vi "graphOnScreen.vi"(6 "Connect to loop iteration":i32, 8 "Time":dbl, 9 "332 Temp [K]":dbl, 10 "332 Temp Setpoint [K]":dbl, 11 "R(ohm)":dbl) -> (0 "T(t)":cluster{"X":dbl, "Y":dbl}[](graph), 3 "?":cluster{dbl, dbl}[](graph))   [LabVIEW 2012]
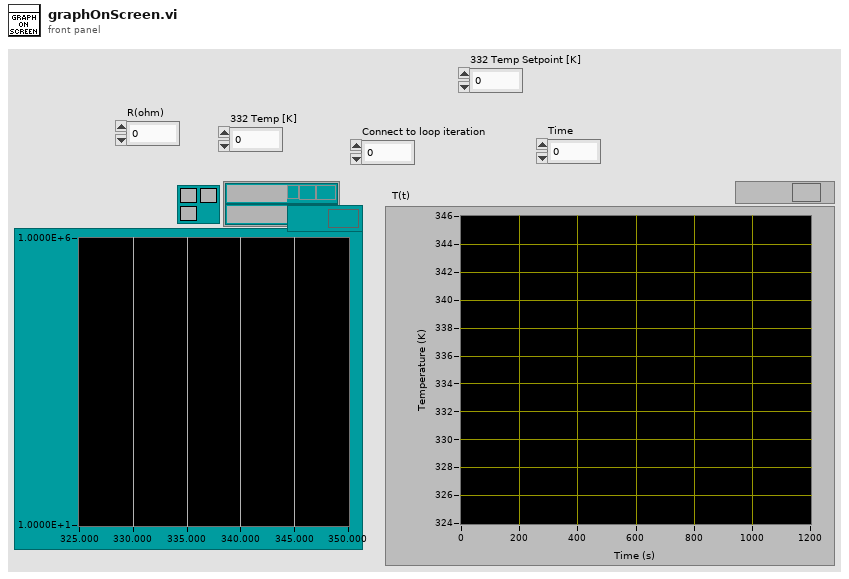
[diagram p1: front panel]
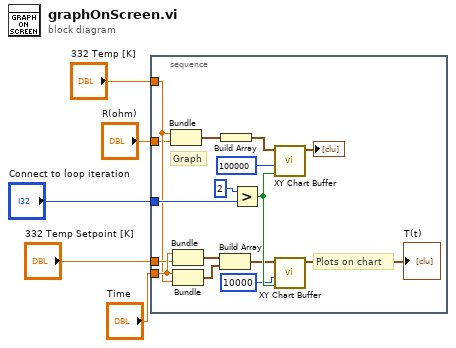
[diagram p0: block diagram]
diagram:
  n1 = stacked-sequence {
    tunnel: "Connect to loop iteration" -> [w17]
    tunnel: "R(ohm)" -> [w6]
    tunnel: "332 Temp [K]" -> [w7]
    tunnel: "Time" -> [w15]
    tunnel: "332 Temp Setpoint [K]" -> [w14]
    frame #0 {
      # "Plots on chart"
      # "Graph"
      n2 = Bundle("332 Temp [K]"=w7, "R(ohm)"=w6) -> (w21:cluster{"332 Temp [K]":dbl, "R(ohm)":dbl})  [unwired: 1 in]
      n3 = Bundle("Time"=w15, "332 Temp Setpoint [K]"=w14) -> (w13:cluster{"Time":dbl, "332 Temp Setpoint [K]":dbl})  [unwired: 1 in]
      n4 = Bundle("Time"=w15, "332 Temp [K]"=w7) -> (w8:cluster{"Time":dbl, "332 Temp [K]":dbl})  [unwired: 1 in]
      n5 = Build Array(w13, w8) -> (w10:cluster{"Time":dbl, "332 Temp [K]":dbl}[])
      n6 = Build Array(w21) -> (w19:cluster{"332 Temp [K]":dbl, "R(ohm)":dbl}[])
      n7 = Greater?(x=2, y=w17) -> (0:w12:bool)
      n8 = call "XY Chart Buffer.vi"("clear first (no:F)"=w12, "chart length (points)"=100000, "new points"=w19) -> ("XY chart data"=→"?":cluster{"x":dbl, "y":dbl}[])  [unwired: 8 in]
      n9 = call "XY Chart Buffer.vi"("clear first (no:F)"=w12, "chart length (points)"=10000, "new points"=w10) -> ("XY chart data"=→"T(t)":cluster{"x":dbl, "y":dbl}[])  [unwired: 8 in]
    }
  }
